vi "YAV_90132_SET_TS.vi"(1 "Address":u8, 2 "Relay Num":u32=2, 3 "error in (no error)":errorcluster, 4 "State":bool) -> (5 "error out":errorcluster)   [LabVIEW 2018]
uses:
  <instrlib>/Phi6/Common/Instrum/Phi6 Core/YAV-System.llb/YAV Card Total Info.ctl
  <instrlib>/Phi6/Common/Instrum/Phi6 Core/YAV-System.llb/YAV Info.ctl
  <instrlib>/Phi6/Common/Instrum/Phi6 Core/YAV-90132.llb/YAV90132 Type Action.ctl
  <instrlib>/Phi6/Common/Instrum/Phi6 Core/YAV-90132.llb/YAV90132 Mode Action.ctl
  <instrlib>/Phi6/Common/Instrum/Phi6 Core/CANNOU Global Variables.llb/CANNOU Global Variables.gbl.vi
panel:
  out "Numeric":i32
  out "Module":T1=enum."YAV90132"
  in  "Info In":T2 {"Version" format="%.0x"; "Options" format="%.0x"; "Index" format="%.0x"}
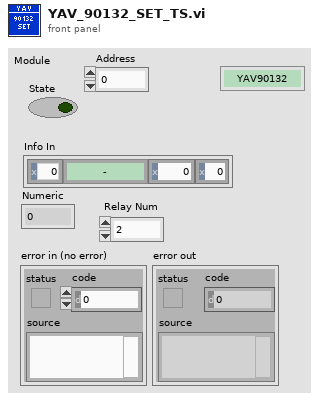
[diagram p1: front panel]
types:
  T1 = typedef "YAV Info.ctl" = enum16{"-", "YAV90832", "YAV904X8", "YAV90132", "YAV91616", "YAV90PIN", "YAV90096", "YAV90HVT", "YAV90CLR", "YAV90128", "YAV90PNE", "YAVCANCON", "YAV91775", "YAV90XXX", "YAV90MMU", "H730050", "H710060", "H710061", "YAV90304", "MMI", "YAV90060", "YAV90MUX", "YAV90059", "YAV90070", "AK087", "Not Defined"}
  T2 = typedef "YAV Card Total Info.ctl" = cluster{"Index":u8, "Module":T1, "Version":u16, "Options":u8}
  T3 = typedef "Module CAN.ctl" = enum16{"CAN0", "CAN1", "CAN2", "CAN3", "CAN4", "CAN5"}
  T4 = typedef "YAV90132 Type Action.ctl" = enum16{"None", "Set OFF", "Set ON", "TOGGLE", "BLINK", "PULSE ON", "PULSE OFF", "ASK", "Set OUT"}
  T5 = typedef "YAV90132 Mode Action.ctl" = enum16{"None", "One Relay", "Several Relays"}
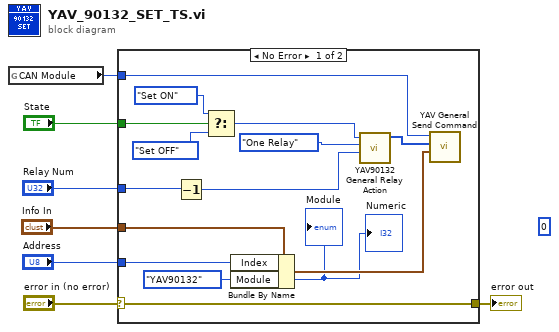
[diagram p0: block diagram]
diagram:
  (unwired) 0
  n1 = global read "CANNOU Global Variables.gbl.vi" "CAN Module"() -> (w1:T3)
  n2 = case shown="No Error" "error in (no error)" {
    selector: "error in (no error)" -> [w9 w22]
    tunnel: "State" -> [w18 _]
    tunnel: w1 -> [w17 _]
    tunnel: "Info In" -> [w14 _]
    tunnel: "Address" -> [w12 _]
    tunnel: "Relay Num" -> [w11 _]
    tunnel: [w9 w22] -> w2
    frame No Error {
      w8 = YAV_Info."YAV90132" ("Module")
      n3 = Decrement(x=w11) -> (x-1=w10:u32)
      n4 = Select(t=YAV90132_Type_Action."Set ON" ("Type Action"), s=w18, f=YAV90132_Type_Action."Set OFF") -> (s? t:f=w21:T4)
      n5 = Bundle By Name(cluster=w14, "Index"=w12, "Module"=w8) -> (w13:T2)
      n6 = call <instrlib>:"YAV90132 General Relay Action.vi"("Relay/Relays"=w10, "Mode Action"=YAV90132_Mode_Action."One Relay", "Type Action"=w21) -> ("Data"=w16:u8[])  [unwired: 8 in]
      n7 = call <instrlib>:"YAV General Send Command.vi"("Info In"=w13, "Data"=w16, "CAN Module"=w17) -> ()  [unwired: 3 in, 2 out]
      "Module" <- w8
      "Numeric" <- w8
    }
    frame Error {
    }
  }
  "error out" <- w2
